vi "SigInfo Init.vi"(8 "error in (no error)":errorcluster) -> (0 "error out":errorcluster, 3 "mzInfo out":refnum<class "SigInfo.lvclass">)   [LabVIEW 2018, in "SigInfo.lvclass"]
uses:
  SigInfo.lvclass
  SigInfo.lvclass/SigInfo.ctl
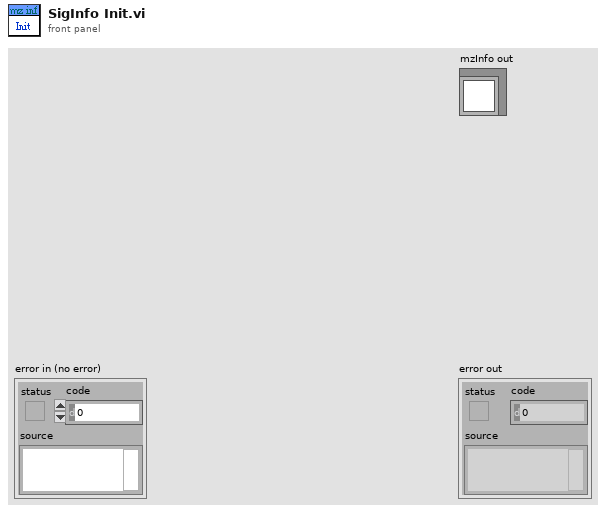
[diagram p1: front panel]
types:
  T1 = cluster{"mzID":u64, "SignalInfo":cluster{"Label":string, "dt":dbl, "Length":u32, "RefVolt":dbl, "mzTable":cluster{"t":dbl[], "mz":dbl[], "beta":dbl[]}}[]}
  T2 = typedef "Semaphore RefNum" = refnum<k1>
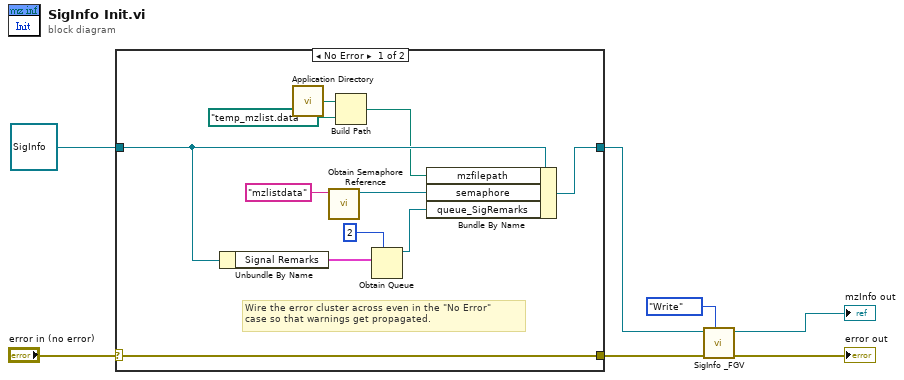
[diagram p0: block diagram]
diagram:
  n1 = case shown="No Error" "error in (no error)" {
    selector: "error in (no error)" -> [w18 w20]
    tunnel: [w18 w20] -> w3
    tunnel: [w15 w19] -> w5
    tunnel: refnum<class "SigInfo.lvclass"> refnum ("mzInfo in") -> [w13 w19]
    frame No Error {
      # "Wire the error cluster across even in the \"No Error\"\ncase so that warnings get propagated."
      n2 = Unbundle By Name(w13) -> ("Signal Remarks"=w14:T1)
      n3 = call <vilib>:"Application Directory.vi"() -> ("Application Directory"=w11:path)
      n4 = call <vilib>:"Obtain Semaphore Reference.vi"("name (unnamed)"="mzlistdata") -> ("semaphore"=w16:T2)  [unwired: 4 in, 2 out]
      n5 = Build Path(base path=w11, name or relative path=path "temp_mzlist.data") -> (appended path=w9:path)
      n6 = Obtain Queue(max queue size (-1, unlimited)=2, element data type=w14) -> (queue out=w8:refnum<queue>)  [unwired: 3 in, 2 out]
      n7 = Bundle By Name(cluster=w13, "mzfilepath"=w9, "semaphore"=w16, "queue_SigRemarks"=w8) -> (w15:refnum<class "SigInfo.lvclass">)
    }
    frame Error {
    }
  }
  n8 = call "SigInfo _FGV.vi"("Function (Read)"=enum16{"Read", "Write"}."Write", "error in (no error)"=w3, "mzInfo in"=w5) -> ("error out"=→"error out":errorcluster, "mzInfo out"=→"mzInfo out":refnum<class "SigInfo.lvclass">)  [unwired: 7 in]
